vi "RPM Analyze.vi"(11 "RPM Data":cluster{"data":dbl[]}[](array[cluster])) -> (2 "Mean RPM":dbl format="%#_13g", 3 "Output XY Graph":cluster{"X":dbl, "Y":dbl}[](array[cluster]))   [LabVIEW 2017]
doc: "This VI converts the number of pulses as measured by the frequency counter to RPM graph that can be sent to Main FP.\n\nThere are a lot of math going on here, but the important one is that there are 360 pulses per revolution (as per spec of the torque transducer) and there are 60 seconds per minute. The frequency counter measures in pulses per second and we need revolutions per minute."
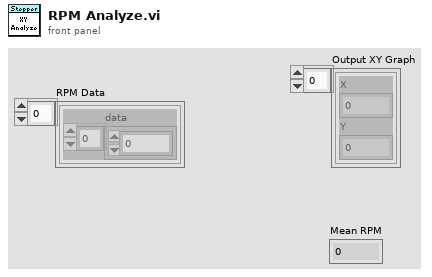
[diagram p1: front panel]
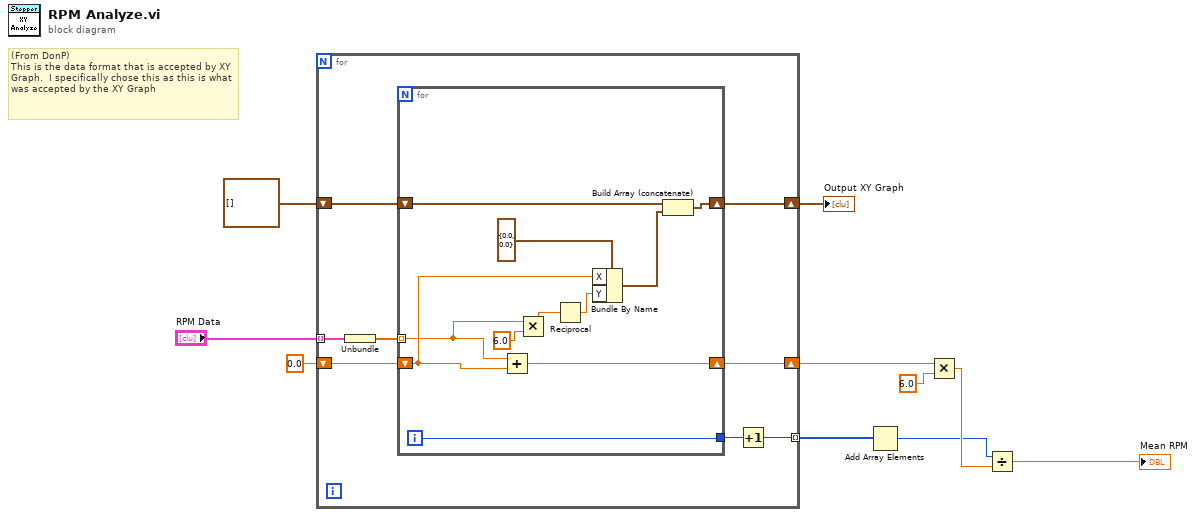
[diagram p0: block diagram]
diagram:
  # "(From DonP)\nThis is the data format that is accepted by XY Graph.  I specifically chose this as this is what was accepted by the XY Graph"
  n1 = for {
    tunnel: "RPM Data" -> [w18] mode=indexing
    shift-right: [w15] -> w3
    shift-left: 0.0 -> [w16]
    shift-right: [w13] -> w7
    shift-left: cluster{"X":dbl, "Y":dbl}[] [] ("Output XY Graph") -> [w14]
    tunnel: [w11] -> w6 mode=indexing
    n2 = Unbundle(w18) -> ("data"=w17:dbl[])
    n3 = for {
      tunnel: w17 -> [w24] mode=indexing
      shift-right: [w29] -> w15
      shift-left: w16 -> [w27]
      shift-right: [w20] -> w13
      shift-left: w14 -> [w22]
      tunnel: [w19] -> w12
      i -> [w19]
      n4 = Add(x=w24, y=w27) -> (x+y=w29:dbl)
      n5 = Multiply(x=w24, y=6.0) -> (x*y=w26:dbl)
      n6 = Reciprocal(x=w26) -> (1/x=w23:dbl)
      n7 = Bundle By Name(cluster=cluster{"X":dbl, "Y":dbl} {"X"=0.0, "Y"=0.0}, "X"=w27, "Y"=w23) -> (w21:cluster{"X":dbl, "Y":dbl})
      n8 = Build Array (concatenate)(w22, w21) -> (w20:cluster{"X":dbl, "Y":dbl}[])
    }
    n9 = Increment(x=w12) -> (x+1=w11:i32)
  }
  "Output XY Graph" <- w7
  n10 = Add Array Elements(numeric array=w6) -> (sum=w2:i32)
  n11 = Multiply(x=w3, y=6.0) -> (x*y=w4:dbl)
  n12 = Divide(x=w2, y=w4) -> (x/y=→"Mean RPM":dbl)
